vi "Barcode(SN)Single.vi"(8 "Button-OK":bool, 10 "menu reference":refnum<k9>, 11 "Barcode(S/N):":string) -> (1 "MainProcess":T1, 3 "Barcode out:":string)   [LabVIEW 2013]
uses:
  Control/SystemProcess.ctl
panel:
  in  "Button-Cancel":bool
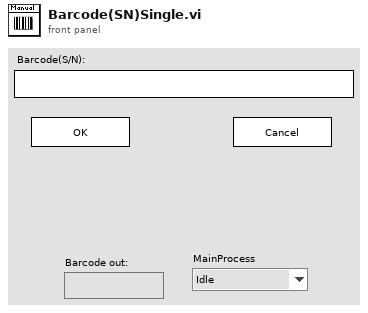
[diagram p1: front panel]
types:
  T1 = typedef "SystemProcess.ctl" = enum16{"Idle", "SystemInit", "SpecialEvent", "Barcode(SN)", "TestInitialize", "Test", "Stop", "SaveTestData", "Exit"}
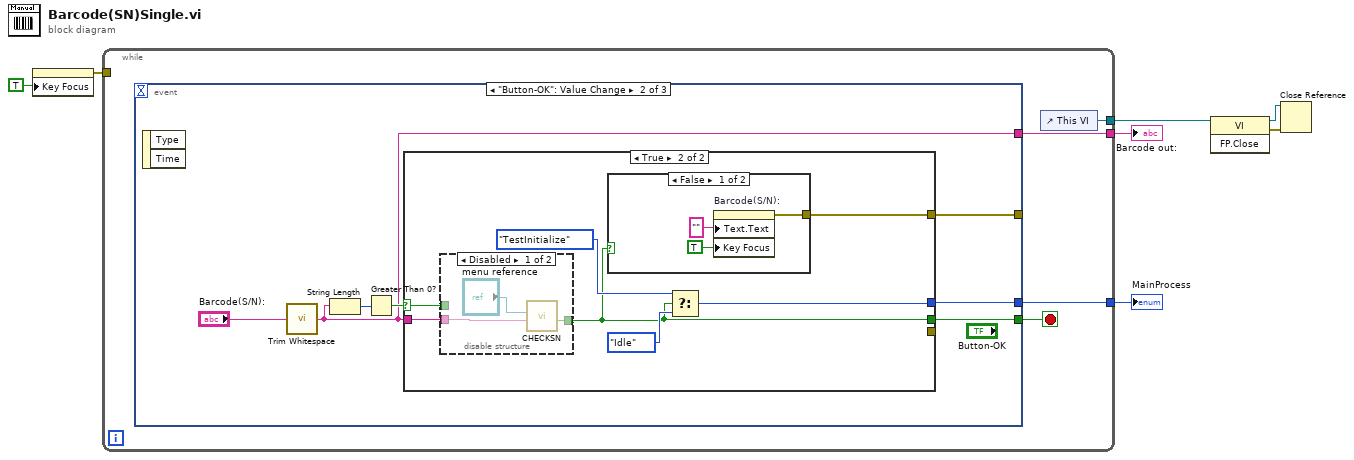
[diagram p0: block diagram]
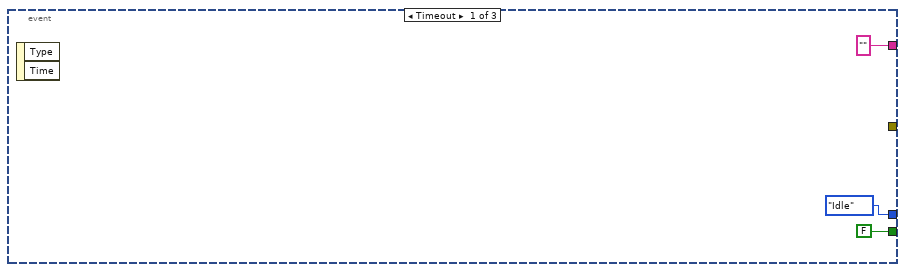
[diagram p2: hidden frame]
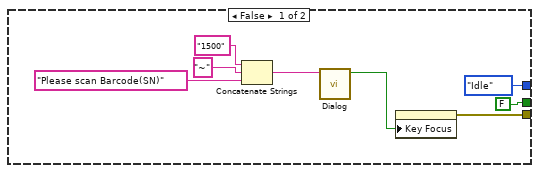
[diagram p3: hidden frame]
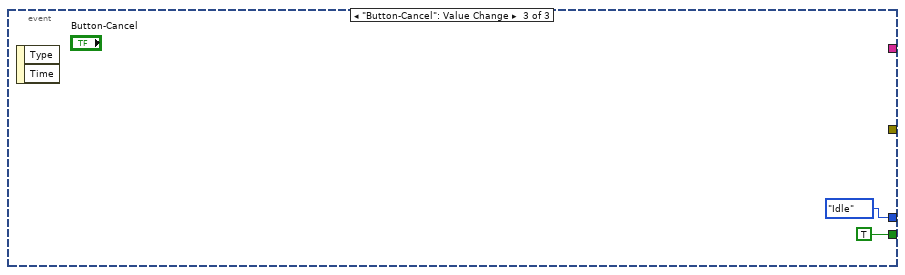
[diagram p6: hidden frame]
diagram:
  n1 = property on="Barcode(S/N):" class="Str"("Key Focus"=TRUE) -> (error out=w2:errorcluster)  [unwired: 2 in, 1 out]
  n2 = while {
    tunnel: [w11] -> w4
    tunnel: [w10] -> w3
    tunnel: w2 -> [_]
    tunnel: [w8] -> w1
    stop <- w9 stop-if-true
    n3 = event shown="[1] \"Button-OK\": Value Change" {
      selector: _ -> [_ _ _]
      dyn-events: _ -> [_ _ _]
      timeout: _ -> [_ _ _]
      tunnel: [FALSE ("OK in") w18 TRUE ("OK in")] -> w9
      tunnel: ["" ("Barcode:") w15 _] -> w10
      tunnel: [SystemProcess."Idle" ("MainProcess") w21 SystemProcess."Idle" ("MainProcess")] -> w8
      tunnel: [_ w17 _] -> _
      event Timeout {
        n4 = event-data() -> ()  [unwired: 1 in, 2 out]
      }
      event "Button-OK": Value Change {
        n5 = event-data() -> ()  [unwired: 1 in, 2 out]
        n6 = call <vilib>:"Trim Whitespace.vi"("string"="Barcode(S/N):") -> ("trimmed string"=w15:string)  [unwired: 1 in]
        n7 = String Length(string=w15) -> (length=w20:i32)
        n8 = Greater Than 0?(x=w20) -> (x > 0?=w19:bool)
        n9 = case shown="True" w19 {
          selector: w19 -> [_ w30]
          tunnel: [SystemProcess."Idle" ("MainProcess") w34] -> w21
          tunnel: [FALSE ("OK in") w32] -> w18
          tunnel: [w27 _] -> _
          tunnel: w15 -> [_ w36]
          tunnel: [_ w31] -> w17
          frame False {
            n10 = Concatenate Strings("1500" ("string"), "~" ("string"), "Please scan Barcode(SN)" ("message")) -> (w23:string)
            n11 = call "Dialog.vi"("Limit"=w23) -> ("true"=w22:bool)  [unwired: 9 in, 1 out]
            n12 = property on="Barcode(S/N):" class="Str"("Key Focus"=w22) -> (error out=w27:errorcluster)  [unwired: 2 in, 1 out]
          }
          frame True {
            n13 = disable-structure shown="Disabled" {
              disable-tunnel: w36 -> [w39 _]
              disable-tunnel: [w37 w40] -> w32
              disable-tunnel: w30 -> [_ w40]
              frame Disabled {
                n14 = call "CHECKSN.vi"("SN"=w39, "menu reference"="menu reference") -> ("SNCheck"=w37:bool)  [unwired: 9 in]
              }
              frame Enabled {
              }
            }
            n15 = case shown="False" w32 {
              tunnel: [w41 _] -> w31
              frame False {
                n16 = property on="Barcode(S/N):" class="Str"("Text.Text"="", "Key Focus"=TRUE) -> (error out=w41:errorcluster)  [unwired: 2 in, 1 out]
              }
              frame True {
              }
            }
            n17 = Select(t=SystemProcess."TestInitialize" ("MainProcess"), s=w32, f=SystemProcess."Idle") -> (s? t:f=w34:T1)
          }
        }
      }
      event "Button-Cancel": Value Change {
        n18 = event-data() -> ()  [unwired: 1 in, 2 out]
      }
    }
    n19 = control-ref of="This VI"() -> (w11:refnum<vi>)
  }
  "Barcode out:" <- w3
  "MainProcess" <- w1
  n20 = invoke class="VI" method="FP.Close"(reference=w4) -> (reference out=w6:refnum<vi>, error out=w5:errorcluster)  [unwired: 2 in, 1 out]
  n21 = Close Reference(reference=w6, error in (no error)=w5) -> ()  [unwired: 1 out]
